vi "Lake Shore 325 Write Curve.vi"(0 "VISA resource name":refnum<visa-resource-name>) -> ()   [LabVIEW 2019]
doc: "This example VI demonstrates the proper use of the Configure Curve Header and Configure Curve Point VIs. It allows the user to write a curve header, a curve point, of both."
uses:
  Lake Shore 325.lvlib
panel:
  in  "Configure Curve Point\n (F: Don't Configure)":bool
  in  "Configure Curve Header \n(F: Don't Configure)":bool
  in  "Temperature Value (0.0000)":dbl format="%.4f"
  in  "Index (1)":dbl=1.0
  in  "Units Value (0.00000)":dbl format="%.5f"
  in  "Curve Serial Number (\"\")":string
  in  "Curve (21)":dbl=21.0
  in  "Curve Name (\"\")":string
  in  "Limit Value (375.000)":dbl=375.0 format="%.3f"
  in  "Curve Data Format (1:mV/K)":u16(ring)=1 items=["mV/K"=1, "V/K"=2, "Ohms/K"=3, "Log Ohms/K"=4]
  in  "Serial Configuration":T1={"Baud Rate"=9600, "Parity"=1, "Data Bits"=7, "Stop Bits"=10, "Flow Control"=0} {"Flow Control" items=["None", "XON/XOFF", "RTS/CTS", "XON/XOFF & RTS/CTS", "DTR/DSR", "XON/XOFF & DTR/DSR"]; "Stop Bits" items=["1.0"=10, "1.5"=15, "2.0"=20]; "Data Bits" items=["7"=7, "8"=8]; "Parity" items=["None", "Odd", "Even", "Mark", "Space"]; "Baud Rate" items=["300"=300, "600"=600, "1200"=1200, "2400"=2400, "4800"=4800, "9600"=9600, "19200"=19200, "38400"=38400, "57600"=57600]}
  # "© 2006 Lake Shore Cryotronics Inc.  ALL RIGHTS RESERVED."
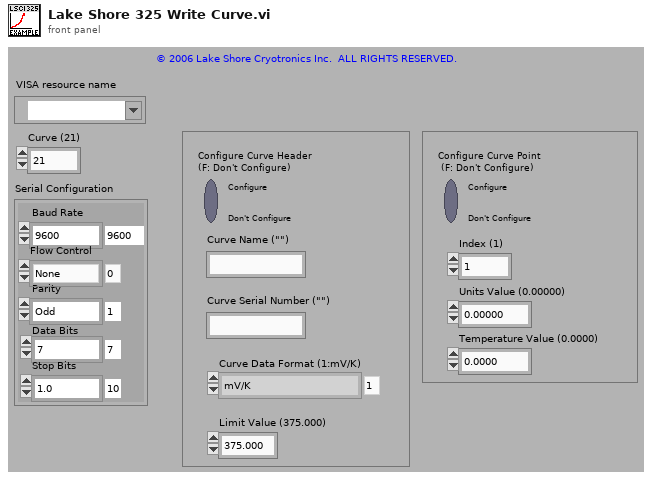
[diagram p1: front panel]
types:
  T1 = cluster{"Baud Rate":u32, "Parity":u16, "Data Bits":u16, "Stop Bits":u16, "Flow Control":u16}
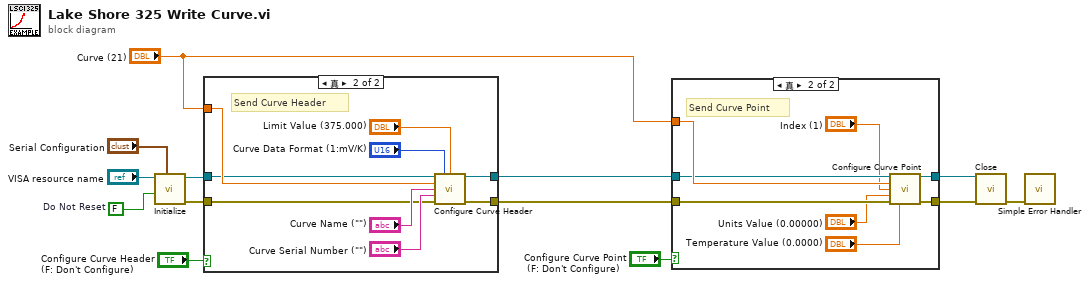
[diagram p0: block diagram]
diagram:
  w10 = FALSE  # Do Not Reset
  n1 = call "Initialize.vi"("Serial Configuration"="Serial Configuration", "Reset (True)"=w10, "VISA resource name"="VISA resource name") -> ("error out"=w7:errorcluster, "VISA resource name out"=w8:refnum<visa-resource-name>)  [unwired: 7 in]
  n2 = case shown="真" "Configure Curve Header \n(F: Don't Configure)" {
    tunnel: "Curve (21)" -> [_ w20]
    tunnel: w8 -> [w15 w19]
    tunnel: w7 -> [w14 w18]
    tunnel: [w15 w17] -> w4
    tunnel: [w14 w16] -> w3
    frame False {
      # "Do Not Send Curve Header"
    }
    frame True {
      # "Send Curve Header"
      n3 = call "Configure Curve Header.vi"("VISA resource name"=w19, "Curve Data Format (1:mV/K)"="Curve Data Format (1:mV/K)", "Limit Value (375.000)"="Limit Value (375.000)", "Curve (21)"=w20, "Curve Name (\"\")"="Curve Name (\"\")", "Curve Serial Number (\"\")"="Curve Serial Number (\"\")", "error in (no error)"=w18) -> ("VISA resource name out"=w17:refnum<visa-resource-name>, "error out"=w16:errorcluster)  [unwired: 7 in]
    }
  }
  n4 = case shown="真" "Configure Curve Point\n (F: Don't Configure)" {
    tunnel: "Curve (21)" -> [_ w34]
    tunnel: w4 -> [w26 w33]
    tunnel: w3 -> [w25 w32]
    tunnel: [w26 w28] -> w2
    tunnel: [w25 w27] -> w1
    frame False {
      # "Do Not Send Curve Point"
    }
    frame True {
      # "Send Curve Point"
      n5 = call "Configure Curve Point.vi"("VISA resource name"=w33, "Curve (21)"=w34, "Index (1)"="Index (1)", "Units Value (0.00000)"="Units Value (0.00000)", "error in (no error)"=w32, "Temperature Value (0.0000)"="Temperature Value (0.0000)") -> ("VISA resource name out"=w28:refnum<visa-resource-name>, "error out"=w27:errorcluster)  [unwired: 8 in]
    }
  }
  n6 = call "Close.vi"("error in (no error)"=w1, "VISA resource name"=w2) -> ("error out"=w11:errorcluster)  [unwired: 9 in]
  n7 = call <vilib>:"Simple Error Handler.vi"("error in (no error)"=w11) -> ()  [unwired: 4 in, 5 out]
